vi "Write MQTTVersion.vi"(10 "MQTTVersion":refnum<class "MQTTVersion.lvclass">, 11 "ControlPacket in":refnum<class "ControlPacket.lvclass">) -> (3 "ControlPacket out":refnum<class "ControlPacket.lvclass">)   [LabVIEW 2013, in "MQTT_Control_Packets.lvlib" / "ControlPacket.lvclass"]
uses:
  ControlPacket.lvclass
  MQTT_311/MQTTVersion.lvclass
  ControlPacket.lvclass/ControlPacket.ctl
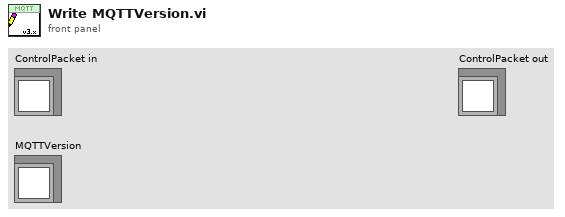
[diagram p1: front panel]
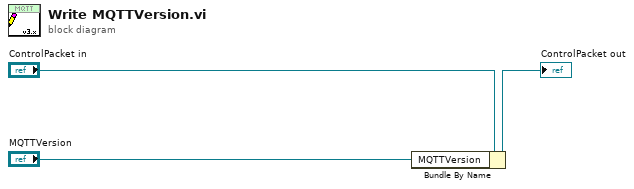
[diagram p0: block diagram]
diagram:
  n1 = Bundle By Name(cluster="ControlPacket in", "MQTTVersion"="MQTTVersion") -> (→"ControlPacket out":refnum<class "ControlPacket.lvclass">)
